vi "DAQ.vi"() -> ()   [LabVIEW 2020]
uses:
  <vilib>/MakerHub/LINX/LMH-LINX.lvlib
  <vilib>/MakerHub/LINX/Public/Peripherals/PWM/PWM Set Duty Cycle 1 Chan.vi
  <vilib>/MakerHub/LINX/Public/Peripherals/Digital/Digital Write N Chans.vi
  <vilib>/MakerHub/LINX/Public/Utilities/Open Serial.vi
panel:
  out "Pression Gauge":dbl[unit](knob)
  out "Thermometer":dbl(slide) scale=0.0..1000.0
  in  "logic":bool[](array[boolean])
  in  "Duty Cycle (0-1)":dbl
  in  "Serial Port":refnum<visa-resource-name>="N/A"
  in  "STOP":bool
  in  "Error In":errorcluster
  # "Control Moteur"
  # "Arduino"
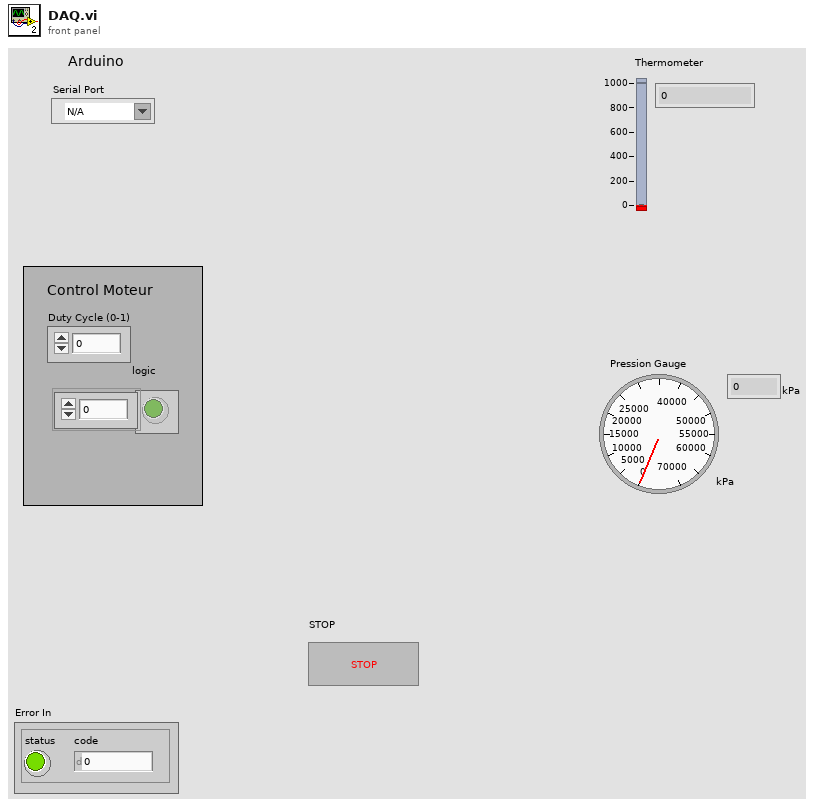
[diagram p1: front panel]
types:
  T1 = typedef "LMH-LINX.lvlib/LINX Ref.ctl" = cluster{"IO":T2, "Interface":T3, "LINX Device Config":T4}
  T2 = typedef "LMH-LINX.lvlib/Platform.ctl" = enum16{"Remote", "Local"}
  T3 = typedef "LMH-LINX.lvlib/Interface.ctl" = enum16{"Serial", "TCP"}
  T4 = typedef "LMH-LINX.lvlib/Device.lvlib/LINX Device Config.ctl" = cluster{"Interface":T3, "COM Port":refnum<visa-resource-name>, "TCP Configuration":T5, "Device Family":u8, "Device ID":u8, "Device Name":string, "TCP Ref":refnum<k5>, "Channels":T6}
  T5 = typedef "LMH-LINX.lvlib/Device.lvlib/TCP Config.ctl" = cluster{"IP Address":string, "Port":u16}
  T6 = typedef "LMH-LINX.lvlib/Channels.ctl" = cluster{"DI":u8[], "DO":u8[], "AI":u8[], "AO":u8[], "PWM":u8[], "QE":u8[], "UART":u8[], "I2C 2":u8[], "SPI":u8[], "CAN":u8[], "Servo":u8[], "AI Ref (V)":dbl, "AI Resolution (Bits)":u8, "AO Ref (V)":dbl, "AO Resolution (Bits)":u8}
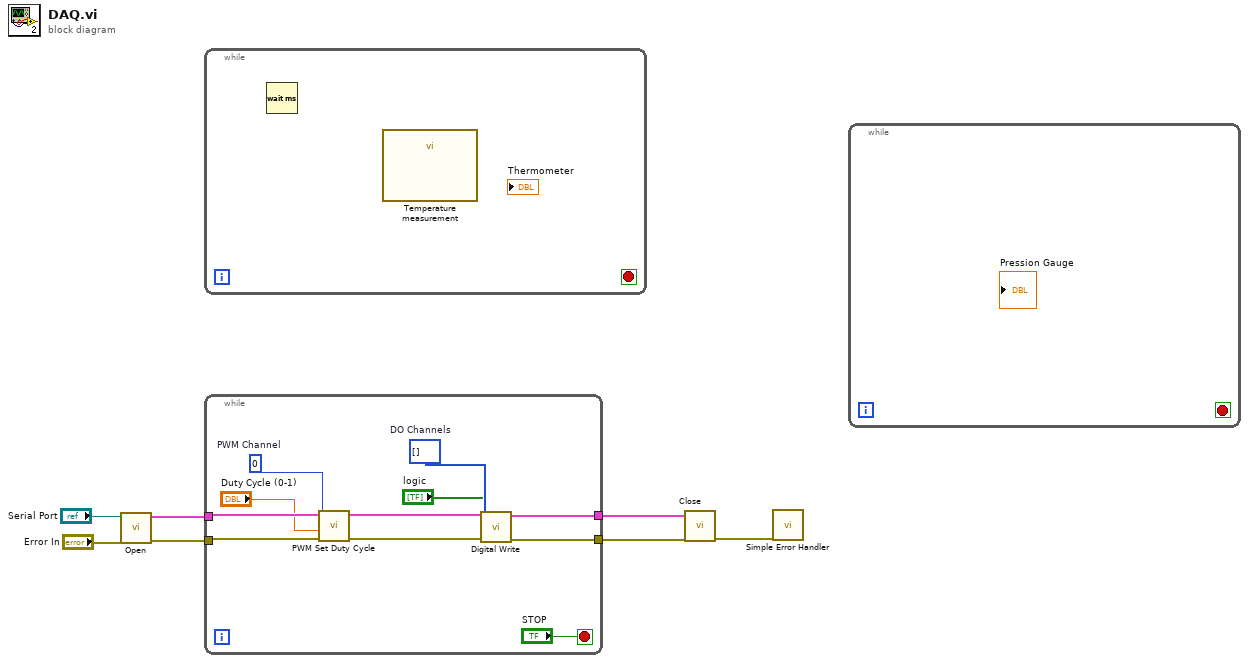
[diagram p0: block diagram]
diagram:
  n1 = call-poly <vilib>:"Open.vi"("Error In"="Error In", "Serial Port"="Serial Port") -> ("Error Out"=w6:errorcluster, "LINX Resource"=w7:T1)  [unwired: 7 in, 1 out]
  n2 = while {
    stop <- _ stop-if-true
    n3 = Wait (ms)() -> ()  [unwired: 1 in, 1 out]
    n4 = call "Temperature measurement"() -> ()  [unwired: 12 in]
  }
  n5 = while {
    tunnel: w7 -> [w18]
    tunnel: w6 -> [w17]
    tunnel: [w12] -> w3
    tunnel: [w11] -> w2
    stop <- "STOP" stop-if-true
    w10 = u8[] []  # DO Channels
    w15 = u8 0  # PWM Channel
    n6 = call-poly <vilib>:"PWM Set Duty Cycle.vi"("Error In"=w17, "Duty Cycle (0-1)"="Duty Cycle (0-1)", "PWM Channel"=w15, "LINX Resource"=w18) -> ("Error Out"=w13:errorcluster, "LINX Resource"=w14:T1)  [unwired: 6 in]
    n7 = call-poly <vilib>:"Digital Write.vi"("Error In"=w13, "Values"="logic", "DO Channels"=w10, "LINX Resource"=w14) -> ("Error Out"=w11:errorcluster, "LINX Resource"=w12:T1)  [unwired: 6 in]
  }
  n8 = call <vilib>:"Close.vi"("Error In"=w2, "LINX Resource"=w3) -> ("Error Out"=w1:errorcluster)  [unwired: 9 in]
  n9 = call <vilib>:"Simple Error Handler.vi"("error in (no error)"=w1) -> ()  [unwired: 4 in, 5 out]
  n10 = while {
    stop <- _ stop-if-true
  }
